vi "HaberlesmeProtek.vi"(6 "Proses":dbl, 7 "VISA resource name":refnum<visa-resource-name>="COM1", 8 "Voltaj set":dbl, 9 "Max.Guc Set":dbl, 10 "Max.Voltaj Set":dbl, 11 "Max.Akım Set":dbl) -> (0 "checked data":bool, 1 "Guc":dbl, 2 "Voltaj":dbl, 3 "Akım":dbl)   [LabVIEW 2016]
panel:
  out "error out":errorcluster
  out "string 5":string
  out "R.checksum":string
  out "aa01xx":string
  out "checksum":string
  out "string 4":string
  out "string 3":string
  out "string":string
  out "string 2":string
  out "Status":bool
  out "substring 7":string
  out "Voltaj Set":dbl
  out "substring 6":string
  out "Max.Guc":dbl
  out "substring 5":string
  out "Max.Voltaj":dbl
  out "substring 4":string
  out "Max.Akım":dbl
  out "substring 3":string
  out "substring 1":string
  out "substring 2":string
  out "Hata mesajı":string
  out "read string":string
  out "Exit":bool
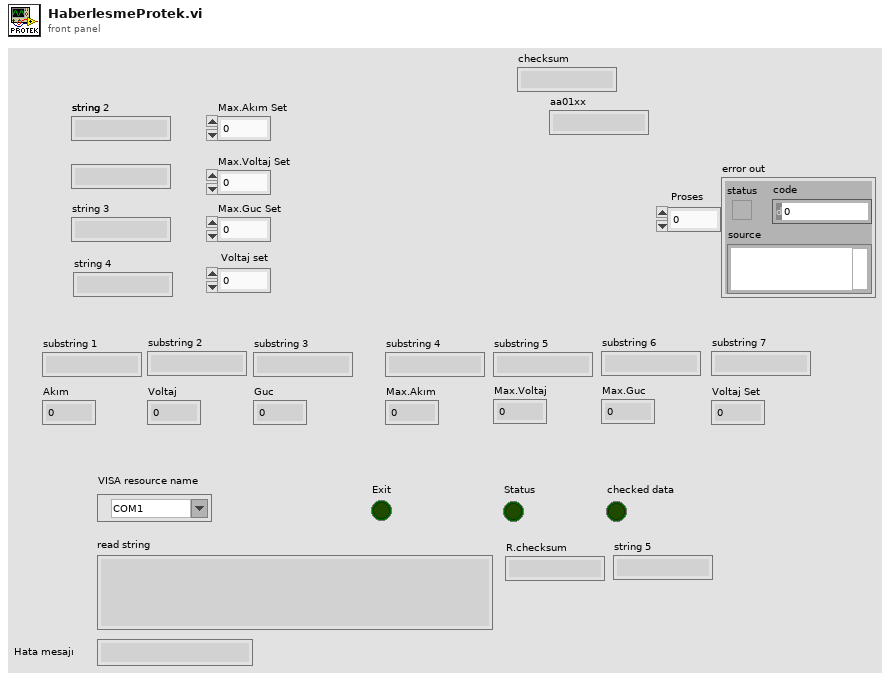
[diagram p1: front panel]
types:
  T1 = enum16{"Start", "Inst recog", "Range read", "Stop"}
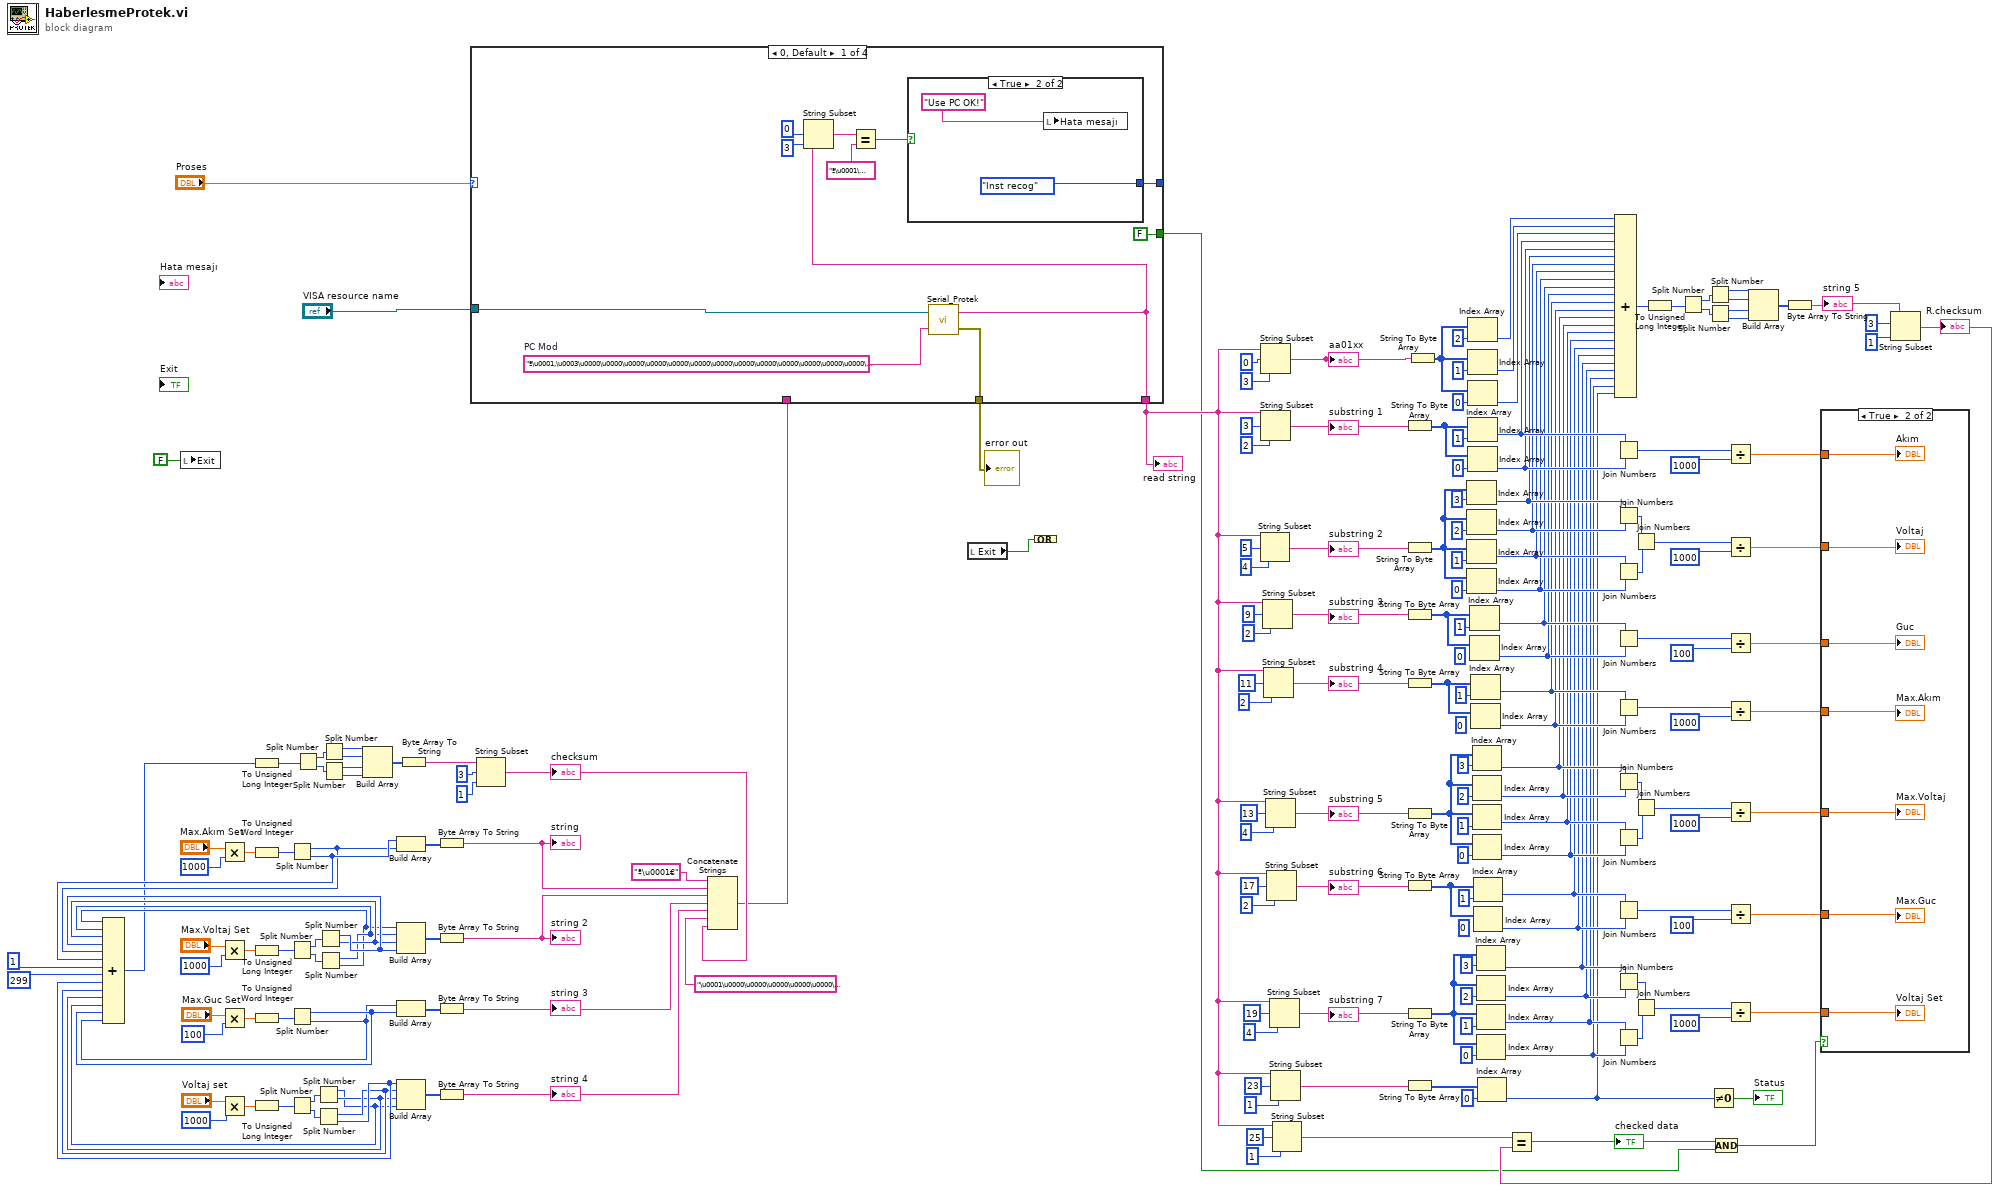
[diagram p0: block diagram]
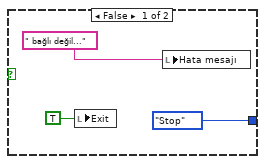
[diagram p3: hidden frame]
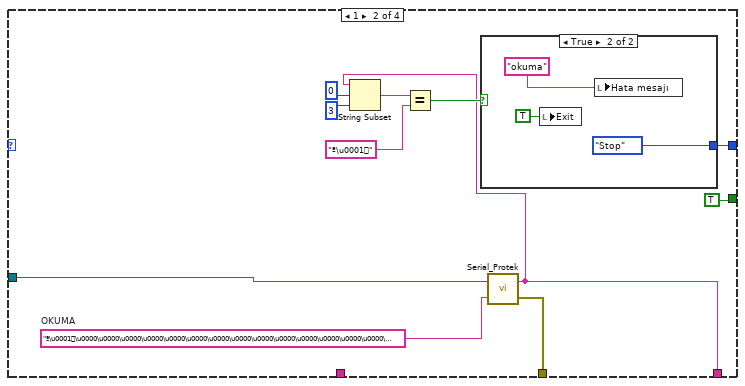
[diagram p4: hidden frame]
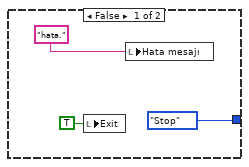
[diagram p5: hidden frame]
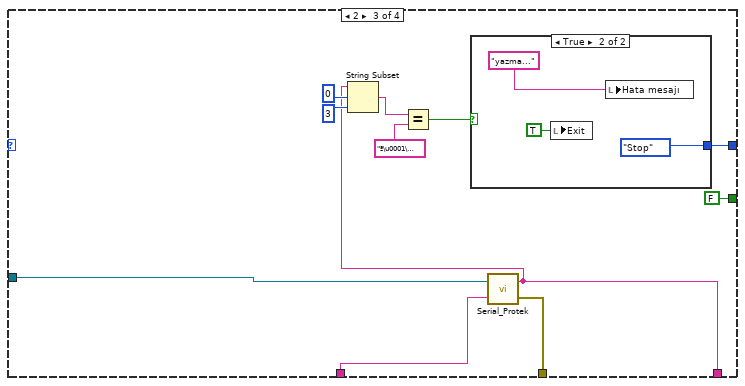
[diagram p6: hidden frame]
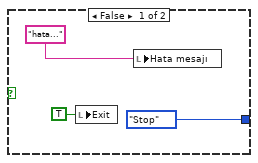
[diagram p7: hidden frame]
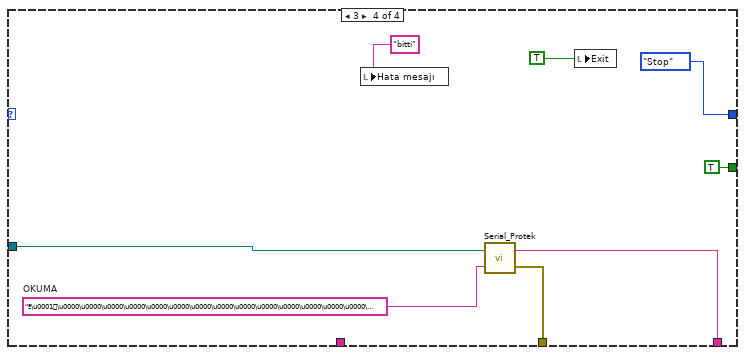
[diagram p8: hidden frame]
diagram:
  (unwired) 0 ("index")
  (unwired) 0 ("index")
  (unwired) 0 ("index")
  n1 = local write "Exit"(FALSE ("Exit")) -> ()
  n2 = Multiply(x="Max.Akım Set", y=u16 1000) -> (x*y=w10:dbl)
  n3 = Multiply(x="Max.Voltaj Set", y=u16 1000) -> (x*y=w14:dbl)
  n4 = Multiply(x="Max.Guc Set", y=u16 100) -> (x*y=w19:dbl)
  n5 = Multiply(x="Voltaj set", y=u16 1000) -> (x*y=w27:dbl)
  n6 = To Unsigned Word Integer(number=w10) -> (unsigned 16bit integer=w11:u16)
  n7 = To Unsigned Long Integer(number=w14) -> (unsigned 32bit integer=w17:u32)
  n8 = To Unsigned Word Integer(number=w19) -> (unsigned 16bit integer=w18:u16)
  n9 = To Unsigned Long Integer(number=w27) -> (unsigned 32bit integer=w24:u32)
  n10 = Split Number(x=w11) -> (hi(x)=w53:u8, lo(x)=w54:u8)
  n11 = Split Number(x=w17) -> (hi(x)=w3:u16, lo(x)=w4:u16)
  n12 = Split Number(x=w18) -> (hi(x)=w59:u8, lo(x)=w46:u8)
  n13 = Split Number(x=w24) -> (hi(x)=w30:u16, lo(x)=w29:u16)
  n14 = Split Number(x=w30) -> (hi(x)=w47:u8, lo(x)=w48:u8)
  n15 = Split Number(x=w29) -> (hi(x)=w49:u8, lo(x)=w50:u8)
  n16 = Split Number(x=w3) -> (hi(x)=w58:u8, lo(x)=w57:u8)
  n17 = Split Number(x=w4) -> (hi(x)=w56:u8, lo(x)=w55:u8)
  n18 = Compound Arithmetic op=unknown(w55, w56, w57, w58, w53, w54, u8 1 ("value"), u16 299 ("value"), w50, w49, w48, w47, w59, w46) -> (w32:u16)
  n19 = To Unsigned Long Integer(number=w32) -> (unsigned 32bit integer=w33:u32)
  n20 = Split Number(x=w33) -> (hi(x)=w34:u16, lo(x)=w35:u16)
  n21 = Split Number(x=w34) -> (hi(x)=w36:u8, lo(x)=w37:u8)
  n22 = Split Number(x=w35) -> (hi(x)=w39:u8, lo(x)=w40:u8)
  n23 = Build Array(w36, w37, w39, w40) -> (w38:u8[])
  n24 = Build Array(w54, w53) -> (w7:u8[])
  n25 = Build Array(w55, w56, w57, w58) -> (w5:u8[])
  n26 = Build Array(w46, w59) -> (w22:u8[])
  n27 = Build Array(w50, w49, w48, w47) -> (w28:u8[])
  n28 = Byte Array To String(unsigned byte array=w38) -> (string=w41:string)
  n29 = Byte Array To String(unsigned byte array=w7) -> (string=w13:string)
  "string" <- w13
  n30 = Byte Array To String(unsigned byte array=w5) -> (string=w12:string)
  "string 2" <- w12
  n31 = Byte Array To String(unsigned byte array=w22) -> (string=w23:string)
  "string 3" <- w23
  n32 = Byte Array To String(unsigned byte array=w28) -> (string=w45:string)
  "string 4" <- w45
  n33 = String Subset(string=w41, offset (0)=3, length (rest)=1 ("length (rest)")) -> (substring=w44:string)
  "checksum" <- w44
  n34 = Concatenate Strings("ª\u0001€" ("element"), w13, w12, w23, w45, "\u0001\u0000\u0000\u0000\u0000\u0000\u0000\u0000\u0000\u0000" ("string"), w44) -> (w2:string)
  n35 = case shown="0, Default" "Proses" {
    tunnel: [w197 w215 w232 T1."Stop"] -> _
    tunnel: "VISA resource name" -> [w196 w214 w231 w247]
    tunnel: [w195 w213 w230 w246] -> w71
    tunnel: [FALSE TRUE FALSE TRUE] -> w61
    tunnel: w2 -> [_ _ w227 _]
    tunnel: [w193 w209 w226 w243] -> w1
    frame 0, Default {
      w203 = "ª\u0001‚\u0003\u0000\u0000\u0000\u0000\u0000\u0000\u0000\u0000\u0000\u0000\u0000\u0000\u0000\u0000\u0000\u0000\u0000\u0000\u0000\u0000\u00000"  # PC Mod
      n36 = call "Serial_Protek.vi"("string to write"=w203, "VISA  name"=w196) -> ("error out"=w193:errorcluster, "read string"=w195:string)
      n37 = String Subset(string=w195, offset (0)=0, length (rest)=3 ("length (rest)")) -> (substring=w198:string)
      n38 = Equal?(x=w198, y="ª\u0001\u0012") -> (x = y?=w201:bool)
      n39 = case shown="True" w201 {
        tunnel: [T1."Stop" T1."Inst recog"] -> w197
        frame False {
          n40 = local write "Exit"(TRUE ("Exit")) -> ()
          n41 = local write "Hata mesajı"(" bağlı değil..." ("Error")) -> ()
        }
        frame True {
          n42 = local write "Hata mesajı"("Use PC OK!" ("Hata mesajı")) -> ()
        }
      }
    }
    frame 1 {
      w210 = "ª\u0001\u0000\u0000\u0000\u0000\u0000\u0000\u0000\u0000\u0000\u0000\u0000\u0000\u0000\u0000\u0000\u0000\u0000\u0000\u0000\u0000\u0000\u0000,"  # OKUMA
      n43 = call "Serial_Protek.vi"("string to write"=w210, "VISA  name"=w214) -> ("error out"=w209:errorcluster, "read string"=w213:string)
      n44 = String Subset(string=w213, offset (0)=0, length (rest)=3 ("length (rest)")) -> (substring=w219:string)
      n45 = Equal?(x=w219, y="ª\u0001") -> (x = y?=w216:bool)
      n46 = case shown="True" w216 {
        tunnel: [T1."Stop" T1."Stop"] -> w215
        frame False {
          n47 = local write "Exit"(TRUE ("Exit")) -> ()
          n48 = local write "Hata mesajı"("hata." ("Error")) -> ()
        }
        frame True {
          n49 = local write "Exit"(TRUE ("Exit")) -> ()
          n50 = local write "Hata mesajı"("okuma" ("Hata mesajı")) -> ()
        }
      }
    }
    frame 2 {
      n51 = call "Serial_Protek.vi"("string to write"=w227, "VISA  name"=w231) -> ("error out"=w226:errorcluster, "read string"=w230:string)
      n52 = String Subset(string=w230, offset (0)=0, length (rest)=3 ("length (rest)")) -> (substring=w233:string)
      n53 = Equal?(x=w233, y="ª\u0001\u0012") -> (x = y?=w229:bool)
      n54 = case shown="True" w229 {
        tunnel: [T1."Stop" T1."Stop"] -> w232
        frame False {
          n55 = local write "Exit"(TRUE ("Exit")) -> ()
          n56 = local write "Hata mesajı"("hata..." ("Hata mesajı")) -> ()
        }
        frame True {
          n57 = local write "Exit"(TRUE ("Exit")) -> ()
          n58 = local write "Hata mesajı"("yazma..." ("Hata mesajı")) -> ()
        }
      }
    }
    frame 3 {
      w244 = "ª\u0001\u0000\u0000\u0000\u0000\u0000\u0000\u0000\u0000\u0000\u0000\u0000\u0000\u0000\u0000\u0000\u0000\u0000\u0000\u0000\u0000\u0000\u0000,"  # OKUMA
      n59 = local write "Hata mesajı"("bitti" ("Hata mesajı")) -> ()
      n60 = call "Serial_Protek.vi"("string to write"=w244, "VISA  name"=w247) -> ("error out"=w243:errorcluster, "read string"=w246:string)
      n61 = local write "Exit"(TRUE ("Start done")) -> ()
    }
  }
  "read string" <- w71
  "error out" <- w1
  n62 = local read "Exit"() -> (w60:bool)
  n63 = Compound Arithmetic op=OR(w60) -> ()  [unwired: 1 out]
  n64 = String Subset(string=w71, offset (0)=5, length (rest)=4 ("length (rest)")) -> (substring=w185:string)
  "substring 2" <- w185
  n65 = String Subset(string=w71, offset (0)=0, length (rest)=3 ("length (rest)")) -> (substring=w116:string)
  "aa01xx" <- w116
  n66 = String Subset(string=w71, offset (0)=3, length (rest)=2 ("length (rest)")) -> (substring=w175:string)
  "substring 1" <- w175
  n67 = String Subset(string=w71, offset (0)=9, length (rest)=2 ("length (rest)")) -> (substring=w165:string)
  "substring 3" <- w165
  n68 = String Subset(string=w71, offset (0)=11, length (rest)=2 ("length (rest)")) -> (substring=w160:string)
  "substring 4" <- w160
  n69 = String Subset(string=w71, offset (0)=13, length (rest)=4 ("length (rest)")) -> (substring=w148:string)
  "substring 5" <- w148
  n70 = String Subset(string=w71, offset (0)=17, length (rest)=2 ("length (rest)")) -> (substring=w141:string)
  "substring 6" <- w141
  n71 = String Subset(string=w71, offset (0)=19, length (rest)=4 ("length (rest)")) -> (substring=w132:string)
  "substring 7" <- w132
  n72 = String Subset(string=w71, offset (0)=23, length (rest)=1 ("length (rest)")) -> (substring=w121:string)
  n73 = String Subset(string=w71, offset (0)=25, length (rest)=1 ("length (rest)")) -> (substring=w73:string)
  n74 = String To Byte Array(string=w175) -> (unsigned byte array=w176:u8[])
  n75 = String To Byte Array(string=w185) -> (unsigned byte array=w182:u8[])
  n76 = String To Byte Array(string=w165) -> (unsigned byte array=w164:u8[])
  n77 = String To Byte Array(string=w160) -> (unsigned byte array=w161:u8[])
  n78 = String To Byte Array(string=w148) -> (unsigned byte array=w151:u8[])
  n79 = String To Byte Array(string=w141) -> (unsigned byte array=w142:u8[])
  n80 = String To Byte Array(string=w132) -> (unsigned byte array=w129:u8[])
  n81 = String To Byte Array(string=w121) -> (unsigned byte array=w120:u8[])
  n82 = String To Byte Array(string=w116) -> (unsigned byte array=w115:u8[])
  n83 = Index Array(array=w182, index=3) -> (element=w106:u8)
  n84 = Index Array(array=w182, index=2) -> (element=w105:u8)
  n85 = Index Array(array=w182, index=1) -> (element=w104:u8)
  n86 = Index Array(array=w182, index=0) -> (element=w103:u8)
  n87 = Index Array(array=w115, index=2) -> (element=w111:u8)
  n88 = Index Array(array=w115, index=1) -> (element=w110:u8)
  n89 = Index Array(array=w115, index=0) -> (element=w109:u8)
  n90 = Index Array(array=w176, index=1) -> (element=w108:u8)
  n91 = Index Array(array=w176, index=0) -> (element=w107:u8)
  n92 = Index Array(array=w164, index=1) -> (element=w102:u8)
  n93 = Index Array(array=w164) -> (element=w101:u8)  [unwired: 1 in]
  n94 = Index Array(array=w161, index=1) -> (element=w100:u8)
  n95 = Index Array(array=w161) -> (element=w99:u8)  [unwired: 1 in]
  n96 = Index Array(array=w151, index=3) -> (element=w98:u8)
  n97 = Index Array(array=w151, index=2) -> (element=w97:u8)
  n98 = Index Array(array=w151, index=1) -> (element=w96:u8)
  n99 = Index Array(array=w151, index=0) -> (element=w95:u8)
  n100 = Index Array(array=w142, index=1) -> (element=w94:u8)
  n101 = Index Array(array=w142) -> (element=w93:u8)  [unwired: 1 in]
  n102 = Index Array(array=w129, index=3) -> (element=w92:u8)
  n103 = Index Array(array=w129, index=2) -> (element=w91:u8)
  n104 = Index Array(array=w129, index=1) -> (element=w90:u8)
  n105 = Index Array(array=w129, index=0) -> (element=w89:u8)
  n106 = Index Array(array=w120, index=0) -> (element=w88:u8)
  n107 = Compound Arithmetic op=ADD(w111, w110, w109, w108, w107, w106, w105, w104, w103, w102, w101, w100, w99, w98, w97, w96, w95, w94, w93, w92, w91, w90, w89, w88) -> (w77:u8)
  n108 = Join Numbers(hi=w108, lo=w107) -> ((hi.lo)=w170:u16)
  n109 = Join Numbers(hi=w106, lo=w105) -> ((hi.lo)=w181:u16)
  n110 = Join Numbers(hi=w104, lo=w103) -> ((hi.lo)=w180:u16)
  n111 = Join Numbers(hi=w102, lo=w101) -> ((hi.lo)=w169:u16)
  n112 = Join Numbers(hi=w100, lo=w99) -> ((hi.lo)=w156:u16)
  n113 = Join Numbers(hi=w98, lo=w97) -> ((hi.lo)=w152:u16)
  n114 = Join Numbers(hi=w96, lo=w95) -> ((hi.lo)=w153:u16)
  n115 = Join Numbers(hi=w94, lo=w93) -> ((hi.lo)=w137:u16)
  n116 = Join Numbers(hi=w92, lo=w91) -> ((hi.lo)=w128:u16)
  n117 = Join Numbers(hi=w90, lo=w89) -> ((hi.lo)=w127:u16)
  n118 = Join Numbers(hi=w181, lo=w180) -> ((hi.lo)=w178:u32)
  n119 = Join Numbers(hi=w152, lo=w153) -> ((hi.lo)=w155:u32)
  n120 = Join Numbers(hi=w128, lo=w127) -> ((hi.lo)=w125:u32)
  n121 = To Unsigned Long Integer(number=w77) -> (unsigned 32bit integer=w85:u32)
  n122 = Split Number(x=w85) -> (hi(x)=w84:u16, lo(x)=w83:u16)
  n123 = Split Number(x=w84) -> (hi(x)=w82:u8, lo(x)=w81:u8)
  n124 = Split Number(x=w83) -> (hi(x)=w79:u8, lo(x)=w78:u8)
  n125 = Not Equal To 0?(x=w88) -> (x != 0?=→"Status":bool)
  n126 = Divide(x=w170, y=u16 1000) -> (x/y=w67:dbl)
  n127 = Divide(x=w178, y=u16 1000) -> (x/y=w66:dbl)
  n128 = Divide(x=w169, y=u16 100) -> (x/y=w65:dbl)
  n129 = Divide(x=w156, y=u16 1000) -> (x/y=w64:dbl)
  n130 = Divide(x=w155, y=u16 1000) -> (x/y=w63:dbl)
  n131 = Divide(x=w137, y=u16 100) -> (x/y=w62:dbl)
  n132 = Divide(x=w125, y=u16 1000) -> (x/y=w70:dbl)
  n133 = Build Array(w82, w81, w79, w78) -> (w80:u8[])
  n134 = Byte Array To String(unsigned byte array=w80) -> (string=w76:string)
  "string 5" <- w76
  n135 = String Subset(string=w76, offset (0)=3, length (rest)=1 ("length (rest)")) -> (substring=w72:string)
  "R.checksum" <- w72
  n136 = Equal?(x=w73, y=w72) -> (x = y?=w69:bool)
  "checked data" <- w69
  n137 = And(x=w69, y=w61) -> (x .and. y?=w68:bool)
  n138 = case shown="True" w68 {
    tunnel: w70 -> [_ w257]
    tunnel: w67 -> [_ w256]
    tunnel: w66 -> [_ w255]
    tunnel: w65 -> [_ w254]
    tunnel: w64 -> [_ w253]
    tunnel: w63 -> [_ w252]
    tunnel: w62 -> [_ w251]
    frame False {
    }
    frame True {
      "Voltaj Set" <- w257
      "Akım" <- w256
      "Voltaj" <- w255
      "Guc" <- w254
      "Max.Akım" <- w253
      "Max.Voltaj" <- w252
      "Max.Guc" <- w251
    }
  }
